vi "Load Tags.vi"(6 "Create Tags? (T)":bool=TRUE, 8 "error in (no error)":errorcluster, 11 "XML File Path":path) -> (0 "error out":errorcluster, 3 "CVT Tags":T1)   [LabVIEW 2016, in "CVT.lvlib" / "Current Value Table.lvlib"]
doc: "This should only be used to load XML files generated by the new CVT. You can still use the old CVT's tag reader on those files."
uses:
  <vilib>/NI/Current Value Table/Current Value Table.lvlib
  <vilib>/NI/Current Value Table/Type Defs/File Format.ctl
  <vilib>/NI/Current Value Table/Type Defs/Single Tag.ctl
  <vilib>/NI/Current Value Table/Type Defs/Data Types.ctl
  <vilib>/NI/Current Value Table/Type Defs/Tag Grouping set.ctl
  <vilib>/Utility/xml.llb/Read From XML File(string).vi
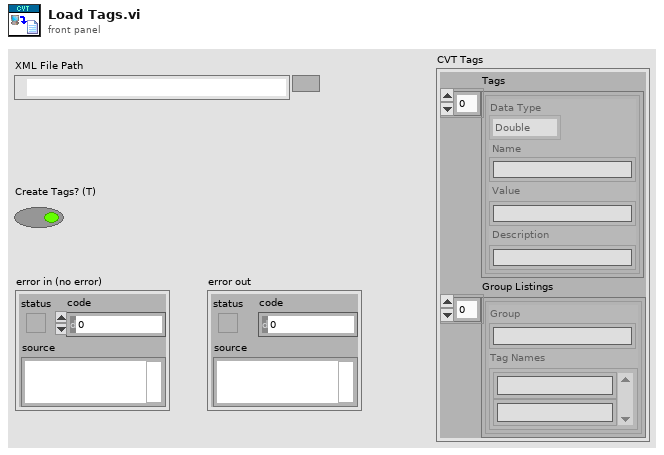
[diagram p1: front panel]
types:
  T1 = typedef "CVT.lvlib/Current Value Table.lvlib/File Format.ctl" = cluster{"Tags":T2[], "Group Listings":T4[]}
  T2 = typedef "CVT.lvlib/Current Value Table.lvlib/Single Tag.ctl" = cluster{"Data Type":T3, "Name":string, "Value":string, "Description":string}
  T3 = typedef "CVT.lvlib/Current Value Table.lvlib/Data Types.ctl" = enum16{"Double", "Single", "I64", "I32", "I16", "I8", "U64", "U32", "U16", "U8", "String", "Boolean", "Array of U8", "Array of U16", "Array of U32", "Array of U64", "Array of I64", "Array of I32", "Array of I16", "Array of I8", "Array of Double", "Array of Single", "Array of Boolean", "Array of String"}
  T4 = typedef "CVT.lvlib/Current Value Table.lvlib/Tag Grouping set.ctl" = cluster{"Group":string, "Tag Names":string[]}
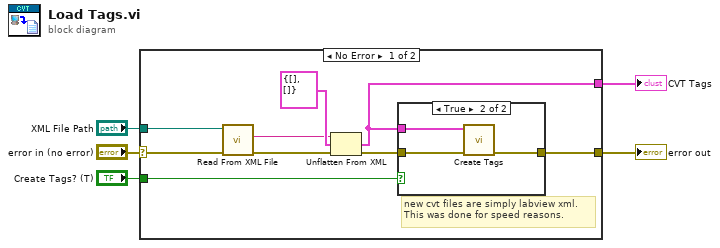
[diagram p0: block diagram]
diagram:
  n1 = case shown="No Error" "error in (no error)" {
    selector: "error in (no error)" -> [w14 w19]
    tunnel: "XML File Path" -> [w13 _]
    tunnel: [w7 w19] -> w3
    tunnel: [w8 _] -> w2
    tunnel: "Create Tags? (T)" -> [w6 _]
    frame No Error {
      # "new cvt files are simply labview xml.\nThis was done for speed reasons."
      n2 = call-poly <vilib>:"Read From XML File.vi"("error in (no error)"=w14, "XML File Path"=w13) -> ("error out"=w12:errorcluster, "XML Elements"=w10:string)  [unwired: 7 in, 1 out]
      n3 = Unflatten From XML(xml string=w10, type=T1 {"Tags"=[], "Group Listings"=[]} ("File Format"), error in (no error)=w12) -> (value=w8:T1, error out=w9:errorcluster)
      n4 = case shown="True" w6 {
        tunnel: w9 -> [w15 w18]
        tunnel: w8 -> [_ w17]
        tunnel: [w15 w16] -> w7
        frame False {
        }
        frame True {
          n5 = call <vilib>:"Create Tags.vi"("error in (no error)"=w18, "CVT Tags to Create"=w17) -> ("error out"=w16:errorcluster)  [unwired: 9 in]
        }
      }
    }
    frame Error {
    }
  }
  "error out" <- w3
  "CVT Tags" <- w2
